vi "CEPMLocalFeedPath.vi"(8 "Error In":errorcluster) -> (0 "Error Out":errorcluster, 3 "CEPM Local Feed Path":path)   [LabVIEW 2019, in "CEPM.lvlib"]
uses:
  <vilib>/Utility/sysdir.llb/System Directory Type.ctl
  CEPM.lvlib
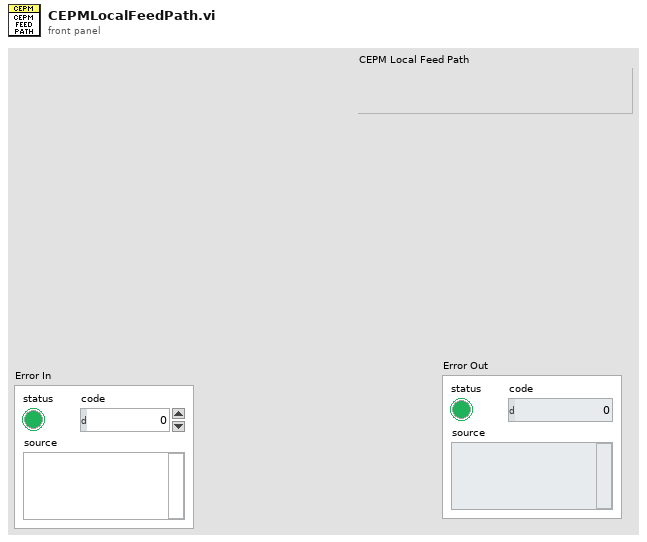
[diagram p1: front panel]
types:
  T1 = typedef "System Directory Type.ctl" = i32
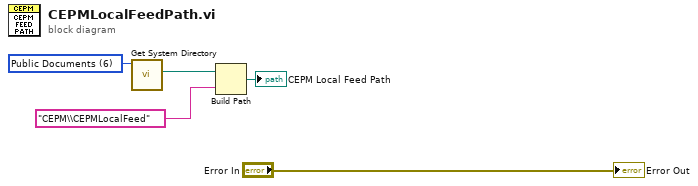
[diagram p0: block diagram]
diagram:
  w5 = T1 6 items=["User Home"=0, "User Desktop"=1, "User Documents"=2, "User Application Data"=3, "User Preferences"=4, "User Temporary"=5, "Public Documents"=6, "Public Application Data"=7, "Public Preferences"=8, "Public Cache"=13, "System Core Libraries"=9, "System Installed Libraries"=10, "Application Files"=11, "Boot Volume Root"=12] ("system directory type")
  n1 = call <vilib>:"Get System Directory.vi"("system directory type"=w5) -> ("system directory"=w4:path)  [unwired: 10 in]
  n2 = Build Path(base path=w4, name or relative path="CEPM\\CEPMLocalFeed") -> (appended path=→"CEPM Local Feed Path":path)
  "Error Out" <- "Error In"
